vi "ev Menu.vi"(8 "error in (no error)":errorcluster, 10 "ItemTag":string, 11 "LF2R IDE in":refnum<class "LF2R IDE.lvclass">) -> (0 "error out":errorcluster, 3 "LF2R IDE out":refnum<class "LF2R IDE.lvclass">)   [LabVIEW 2018, in "LF2R IDE.lvlib" / "LF2R IDE.lvclass"]
uses:
  LF2R IDE.lvclass
  Menu item.ctl
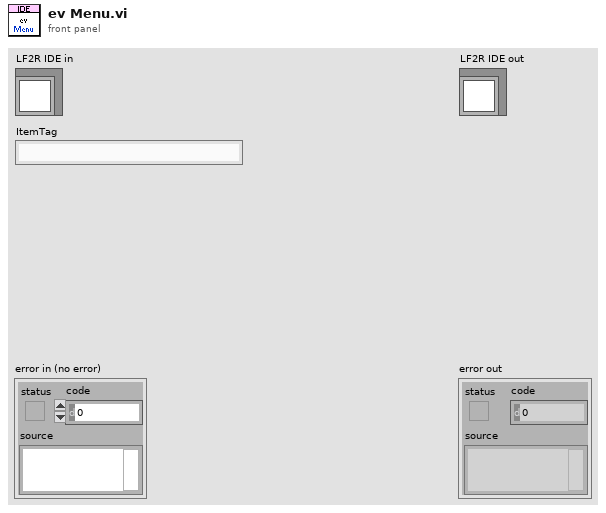
[diagram p1: front panel]
types:
  T1 = typedef "LF2R IDE.lvlib/LF2R IDE.lvclass/Menu Item.ctl" = enum16{"INVALID ITEM", "Open File", "Save File", "Exit", "Preferences"}
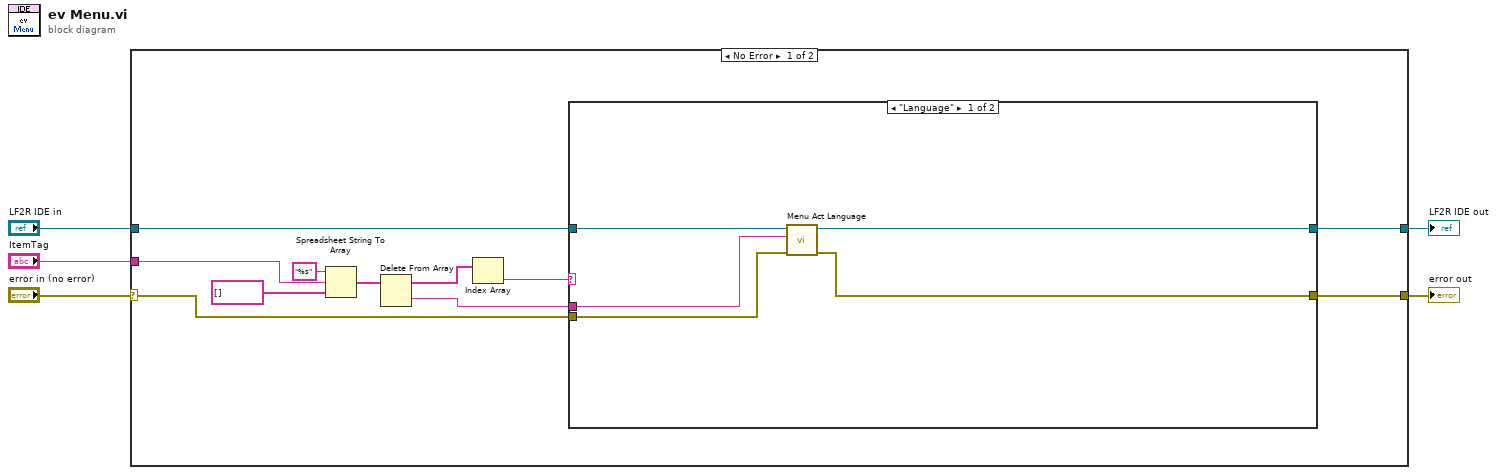
[diagram p0: block diagram]
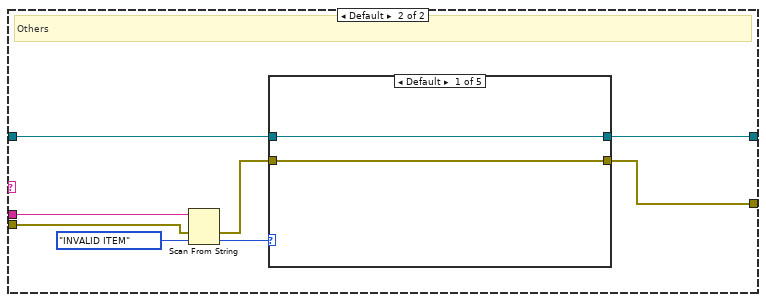
[diagram p2: hidden frame]
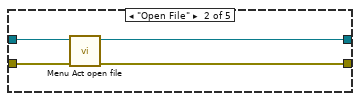
[diagram p3: hidden frame]
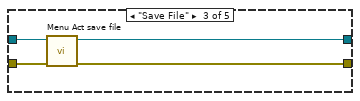
[diagram p4: hidden frame]
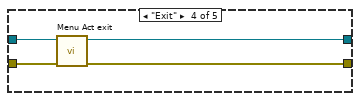
[diagram p5: hidden frame]
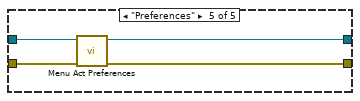
[diagram p6: hidden frame]
diagram:
  n1 = case shown="No Error" "error in (no error)" {
    selector: "error in (no error)" -> [w13 w49]
    tunnel: [w14 w49] -> w4
    tunnel: [w15 w48] -> w2
    tunnel: "LF2R IDE in" -> [w16 w48]
    tunnel: "ItemTag" -> [w12 _]
    frame No Error {
      n2 = Spreadsheet String To Array(format string="%s", spreadsheet string=w12, array type (2D Dbl)=string[] []) -> (array=w9:string[])  [unwired: 1 in]
      n3 = Delete From Array(array=w9) -> (deleted portion=w8:string, array with subset deleted=w7:string[])  [unwired: 2 in]
      n4 = Index Array(array=w7) -> (element=w6:string)  [unwired: 1 in]
      n5 = case shown="\"Language\"" w6 {
        tunnel: w16 -> [w21 w27]
        tunnel: [w20 w25] -> w15
        tunnel: [w19 w24] -> w14
        tunnel: w13 -> [w18 w23]
        tunnel: w8 -> [w17 w22]
        frame "Language" {
          n6 = call "Menu Act Language.vi"("error in (no error)"=w18, "Language Name"=w17, "LF2R IDE in"=w21) -> ("error out"=w19:errorcluster, "LF2R IDE out"=w20:refnum<class "LF2R IDE.lvclass">)  [unwired: 7 in]
        }
        frame Default {
          # "Others"
          n7 = Scan From String(input string=w22, error in=w23, default 1=Menu_Item."INVALID ITEM" ("Menu item")) -> (error out=w26:errorcluster, output 1=w28:T1)  [unwired: 2 in, 2 out]
          n8 = case shown="Default" w28 {
            tunnel: w27 -> [w31 w35 w39 w43 w47]
            tunnel: w26 -> [w30 w34 w38 w42 w46]
            tunnel: [w31 w33 w37 w41 w44] -> w25
            tunnel: [w30 w32 w36 w40 w45] -> w24
            frame Default {
            }
            frame "Open File" {
              n9 = call "Menu Act open file.vi"("error in (no error)"=w34, "LF2R IDE in"=w35) -> ("error out"=w32:errorcluster, "LF2R IDE out"=w33:refnum<class "LF2R IDE.lvclass">)  [unwired: 8 in]
            }
            frame "Save File" {
              n10 = call "Menu Act save file.vi"("error in (no error)"=w38, "LF2R IDE in"=w39) -> ("error out"=w36:errorcluster, "LF2R IDE out"=w37:refnum<class "LF2R IDE.lvclass">)  [unwired: 8 in]
            }
            frame "Exit" {
              n11 = call "Menu Act exit.vi"("error in (no error)"=w42, "LF2R IDE in"=w43) -> ("error out"=w40:errorcluster, "LF2R IDE out"=w41:refnum<class "LF2R IDE.lvclass">)  [unwired: 8 in]
            }
            frame "Preferences" {
              n12 = call "Menu Act Preferences.vi"("error in (no error)"=w46, "LF2R IDE in"=w47) -> ("error out"=w45:errorcluster, "LF2R IDE out"=w44:refnum<class "LF2R IDE.lvclass">)  [unwired: 8 in]
            }
          }
        }
      }
    }
    frame Error {
    }
  }
  "error out" <- w4
  "LF2R IDE out" <- w2
